vi "Print.vi"(8 "error in (no error)":errorcluster, 10 "On?":bool, 11 "Feeder Actor.lvlib:Counter.lvclass":refnum<class "Counter.lvclass">) -> (0 "error out":errorcluster, 3 "Feeder Actor.lvlib:Counter.lvclass 2":refnum<class "Counter.lvclass">)   [LabVIEW 2018, in "Feeder Actor.lvlib" / "Counter.lvclass"]
uses:
  Counter.lvclass
  C:/Program Files/National Instruments/LabVIEW 2018/vi.lib/ActorFramework/Actor/Actor.lvclass
  <vilib>/ActorFramework/Actor/Actor.lvclass/Actor.ctl
  <vilib>/ActorFramework/Message Enqueuer/Message Enqueuer.lvclass/Message Enqueuer.ctl
  Counter.lvclass/Counter.ctl
  <vilib>/ActorFramework/Message Enqueuer/Init from Existing Queue.vi
  <vilib>/ActorFramework/Message Enqueuer/Message Enqueuer.lvclass
  <vilib>/ActorFramework/Actor/Actor.lvclass
  Counter Messages/Set Counter Msg/Set Counter Msg.lvclass
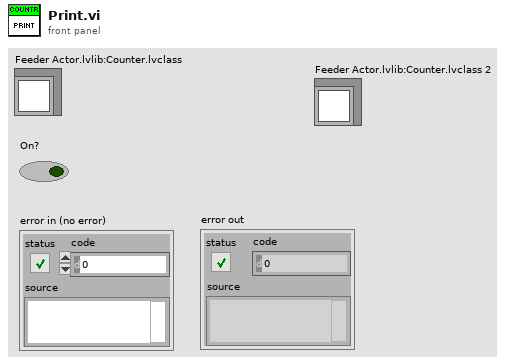
[diagram p1: front panel]
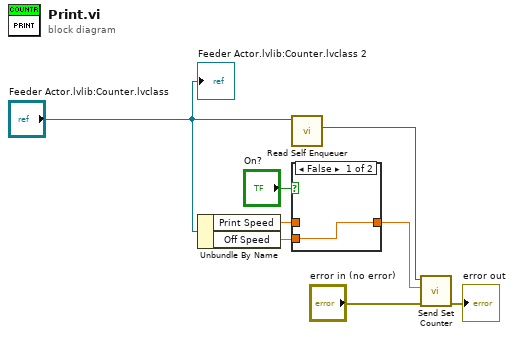
[diagram p0: block diagram]
diagram:
  n1 = Unbundle By Name("Feeder Actor.lvlib:Counter.lvclass") -> ("Print Speed"=w8:dbl, "Off Speed"=w1:dbl)
  n2 = call <vilib>:"Read Self Enqueuer.vi"("Actor"="Feeder Actor.lvlib:Counter.lvclass") -> ("Self Enqueuer"=w2:refnum<class "Message Enqueuer.lvclass">)  [unwired: 10 in]
  n3 = case shown="False" "On?" {
    tunnel: w8 -> [_ w10]
    tunnel: [w9 w10] -> w4
    tunnel: w1 -> [w9 _]
    frame False {
    }
    frame True {
    }
  }
  n4 = call "Send Set Counter.vi"("error in (no error)"="error in (no error)", "Input"=w4, "Message Enqueuer in"=w2) -> ("error out"=→"error out":errorcluster)  [unwired: 7 in, 1 out]
  "Feeder Actor.lvlib:Counter.lvclass 2" <- "Feeder Actor.lvlib:Counter.lvclass"
